vi "2sComplement.vi"(10 "Data In":u32[](array[numeric])) -> (2 "Data Out":i32[](array[numeric]))   [LabVIEW 2014]
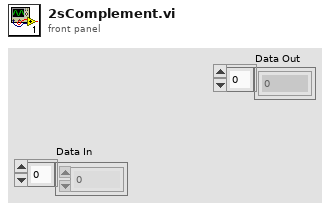
[diagram p1: front panel]
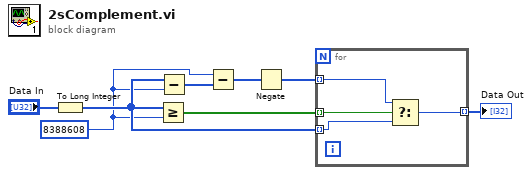
[diagram p0: block diagram]
diagram:
  w3 = 8388608
  n1 = To Long Integer(number="Data In") -> (32bit integer=w5:i32[])
  n2 = Greater Or Equal?(x=w5, y=w3) -> (x >= y?=w8:bool[])
  n3 = Subtract(x=w5, y=w3) -> (x-y=w4:i32[])
  n4 = Subtract(x=w3, y=w4) -> (x-y=w2:i32[])
  n5 = Negate(x=w2) -> (-x=w1:i32[])
  n6 = for {
    tunnel: w8 -> [w12] mode=indexing
    tunnel: w1 -> [w11] mode=indexing
    tunnel: w5 -> [w10] mode=indexing
    tunnel: [w9] -> w7 mode=indexing
    n7 = Select(t=w11, s=w12, f=w10) -> (s? t:f=w9:i32)
  }
  "Data Out" <- w7
